vi "Priority.vi"(8 "error in (no error)":errorcluster, 11 "Caching Request in":refnum<class "Caching Request.lvclass">) -> (0 "error out":errorcluster, 2 "Priority":u16, 3 "Caching Request out":refnum<class "Caching Request.lvclass">)   [LabVIEW 2020, in "HTTP Server.lvlib" / "Caching Request.lvclass"]
uses:
  Caching Request.lvclass
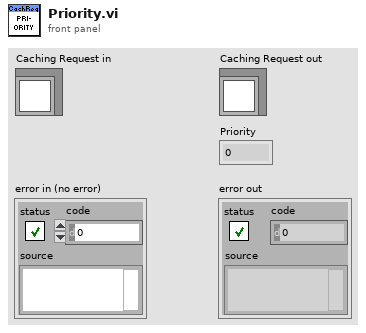
[diagram p1: front panel]
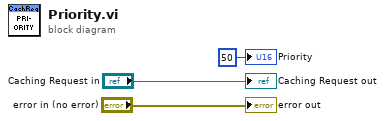
[diagram p0: block diagram]
diagram:
  "error out" <- "error in (no error)"
  "Caching Request out" <- "Caching Request in"
  "Priority" <- u16 50 ("Priority")
